vi "Hex Num Range Array.vi"(8 "error in (no error)":errorcluster, 9 "Check String":string, 10 "HEX_Min":string, 11 "HEX_Max":string="1A") -> (0 "error out":errorcluster, 2 "Check Result":bool, 3 "HEX String":string[](array[string]))   [LabVIEW 2020]
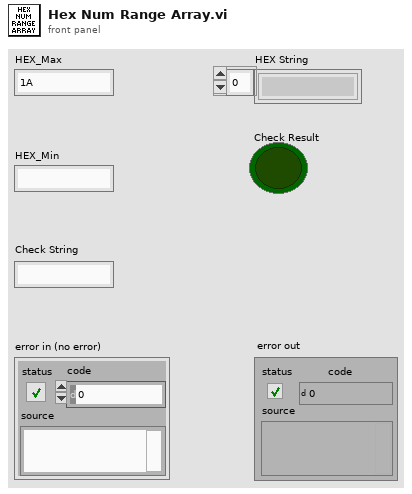
[diagram p1: front panel]
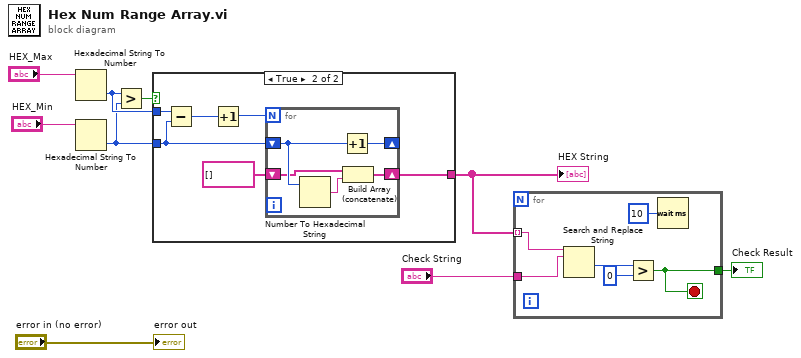
[diagram p0: block diagram]
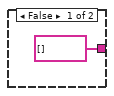
[diagram p2: hidden frame]
diagram:
  n1 = Hexadecimal String To Number(string="HEX_Max") -> (number=w6:u32)  [unwired: 2 in, 1 out]
  n2 = Hexadecimal String To Number(string="HEX_Min") -> (number=w5:u32)  [unwired: 2 in, 1 out]
  n3 = Greater?(x=w6, y=w5) -> (0:w7:bool)
  n4 = case shown="True" w7 {
    tunnel: w6 -> [_ w16]
    tunnel: w5 -> [_ w15]
    tunnel: [string[] [] w13] -> w3
    frame False {
    }
    frame True {
      n5 = Subtract(x=w16, y=w15) -> (x-y=w11:u32)
      n6 = Increment(x=w11) -> (x+1=w12:u32)
      n7 = for {
        N: w12 -> [_]
        shift-right: [w18] -> w13
        shift-left: string[] [] -> [w19]
        shift-right: [w17] -> _
        shift-left: w15 -> [w21]
        n8 = Number To Hexadecimal String(2:w21) -> (0:w20:string)  [unwired: 1 in]
        n9 = Increment(x=w21) -> (x+1=w17:u32)
        n10 = Build Array (concatenate)(w19, w20) -> (w18:string[])
      }
    }
  }
  "HEX String" <- w3
  n11 = for {
    tunnel: w3 -> [w27] mode=indexing
    tunnel: "Check String" -> [w26]
    tunnel: [w23] -> w1
    stop <- w23 stop-if-true
    n12 = Search and Replace String(input string=w27, search string=w26) -> (number of replacements=w25:i32)  [unwired: 6 in, 3 out]
    n13 = Greater?(x=w25, y=0) -> (0:w23:bool)
    n14 = Wait (ms)(milliseconds to wait=u32 10) -> ()  [unwired: 1 out]
  }
  "Check Result" <- w1
  "error out" <- "error in (no error)"
